vi "Handle Click on Tree Item.vi"(5 "Button":u16, 7 "PlatMods":T1, 8 "error in (no error)":errorcluster, 9 "Mods":cluster{"Double Click":bool, "Menu Key":bool}, 10 "Coords":T2, 11 "File Explorer in":refnum<class "File Explorer.lvclass">) -> (0 "error out":errorcluster, 3 "File Explorer out":refnum<class "File Explorer.lvclass">)   [LabVIEW 2020, in "File Explorer.lvlib" / "File Explorer.lvclass"]
doc: "<RequiredOverrideReason>Implement the response to the user left clicking on the tree.</RequiredOverrideReason>"
uses:
  <vilib>/gpm_packages/@cs/file-explorer-extension/Source/File Explorer/File Explorer/File Explorer.lvclass
  <vilib>/Utility/miscctls.llb/LVPoint32TypeDef.ctl
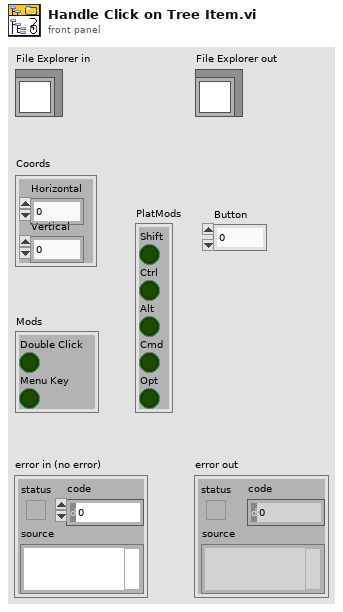
[diagram p1: front panel]
types:
  T1 = cluster{"Shift":bool, "Ctrl":bool, "Alt":bool, "Cmd":bool, "Opt":bool}
  T2 = typedef "LVPoint32TypeDef.ctl" = cluster{"Horizontal":i32, "Vertical":i32}
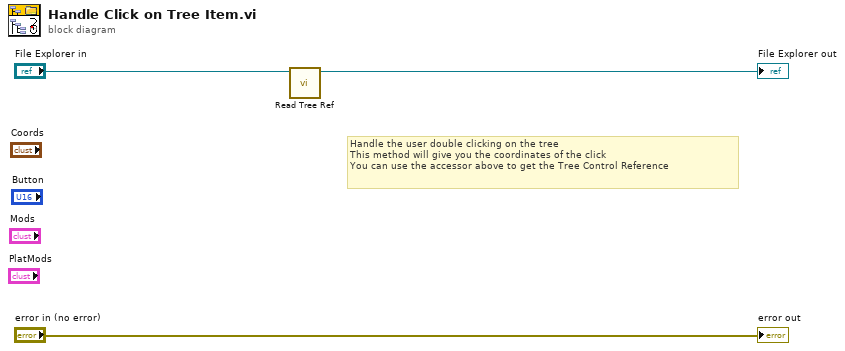
[diagram p0: block diagram]
diagram:
  # "Handle the user double clicking on the tree\nThis method will give you the coordinates of the click\nYou can use the accessor above to get the Tree Control Reference"
  n1 = call <vilib>:"Read Tree Ref.vi"("File Explorer in"="File Explorer in") -> ("File Explorer out"=→"File Explorer out":refnum<class "File Explorer.lvclass">)  [unwired: 8 in, 2 out]
  "error out" <- "error in (no error)"
